vi "FTW-Test-Actor-Stress.vi"() -> (0 "Test Result":errorcluster)   [LabVIEW 2015]
uses:
  src/time/FTW-Time-RelativeTimer.vi
  src/error/FTW-ERR-PrependExplanation.vi
  src/error/FTW-ERR-Ignore.vi
  src/error/FTW-ERR-ThrowError.vi
  src/reflection/FTW-Reflection-Type.vi
  src/error/FTW-ERR-StatusException.vi
  src/error/FTW-ERR-CallChain.vi
  src/string/FTW-STR-ReplaceWhitespace.vi
  src/reflection/FTW-Reflection-Array.vi
  src/error/FTW-ERR-Clear.vi
  src/regex/FTW-Regex-ReplaceAll.vi
  src/json/FTW-JSON-Construct-FromBuffer.vi
  src/json/FTW-JSON-Object-GetElement-String.vi
  src/socket/syncserver/FTW-SyncServer-Construct.vi
  src/json/FTW-JSON-Object-SetElement-String.vi
  src/json/FTW-JSON-Object-GetElement-Bool.vi
  src/json/FTW-JSON-Object-GetElement-Integer.vi
  src/json/FTW-JSON-SerializeAndDestroy.vi
  src/actor/support/FTW-Actor-DynamicLaunchOptions.vi
  src/socket/syncserver/FTW-SyncServer-Await.vi
  src/actor/request/FTW-Request-InterpretResponse.vi
  lib/FTW-KernelFilepath.vi
  src/json/core/FTW-JSON-Core-EncodingFlags.vi
  codegen/xnode/json/fetch/FTW-JSON-Core-GetFlattenedValue.vi
  src/socket/connector/FTW-Connector-Construct.vi
  src/socket/syncserver/FTW-SyncServer-Reply.vi
  src/socket/syncserver/FTW-SyncServer-Destroy.vi
  codegen/xnode/FTW-Dataflow-Synchronizer.xnode
  codegen/xnode/FTW-Actor-Spawn.xnode
  src/core/type/FTW-Type-Actor-Connector.ctl
  codegen/xnode/FTW-JSON-Fetch.xnode
panel:
  out "Actor Lifetimes":dbl[][](graph)
  out "Timeline":cluster{dbl[], i32[]}[](graph)
  in  "Test to Perform":T1(radio)=enum."true 10x10"
  out "Message Times":dbl[][](graph)
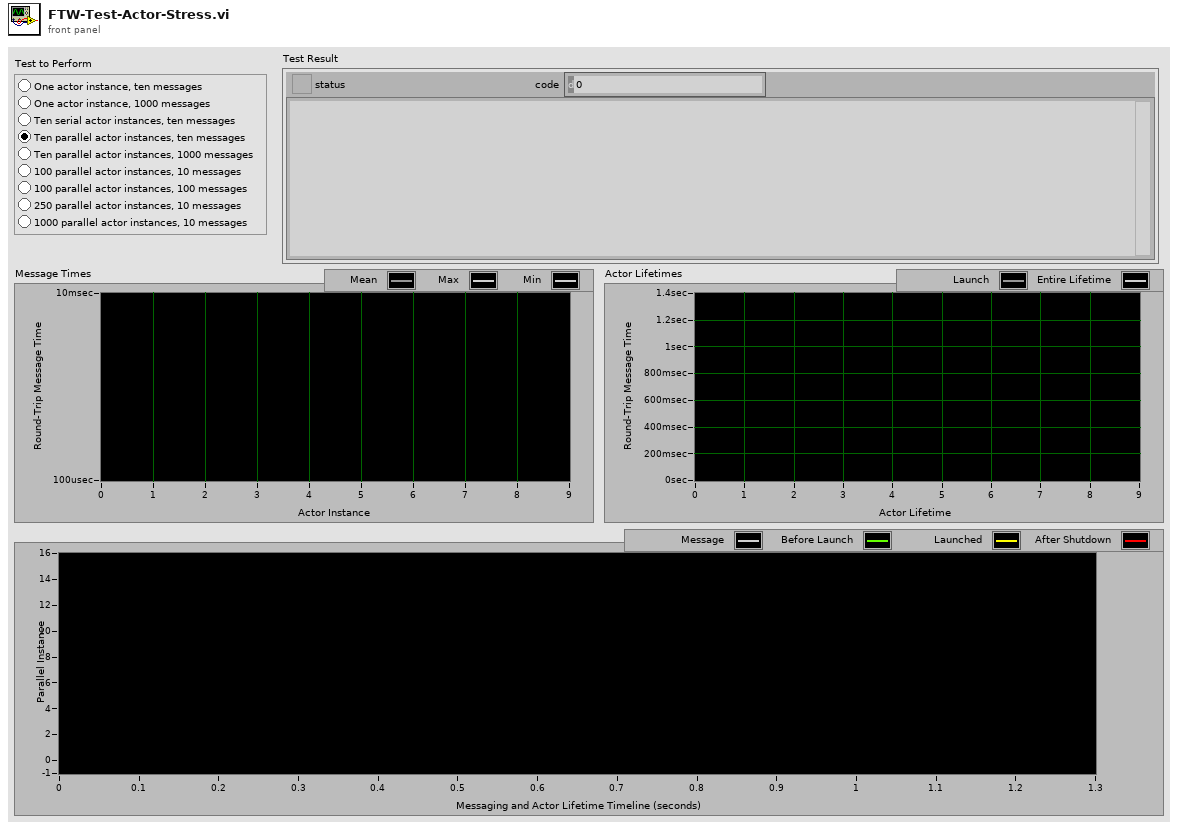
[diagram p1: front panel]
types:
  T1 = enum32{"false 1x10", "false 1x1000", "false 10x10", "true 10x10", "true 10x1000", "true 100x10", "true 100x100", "true 250x10", "true 1000x10"}
  T2 = cluster{"FTW-PrimaryInboxAddress":string, "FTW-InstanceCloneName":string}
  T3 = typedef "FTW-Type-Actor-Connector.ctl" = refnum<data-value>
  T4 = cluster{i32, "High-Resolution Timer":dbl, "Instance Inbox Address":string, "Instance VI Clone Name":string, "High-Resolution Timer":dbl, dbl[], dbl[], "High-Resolution Timer":dbl, "error out out":errorcluster}
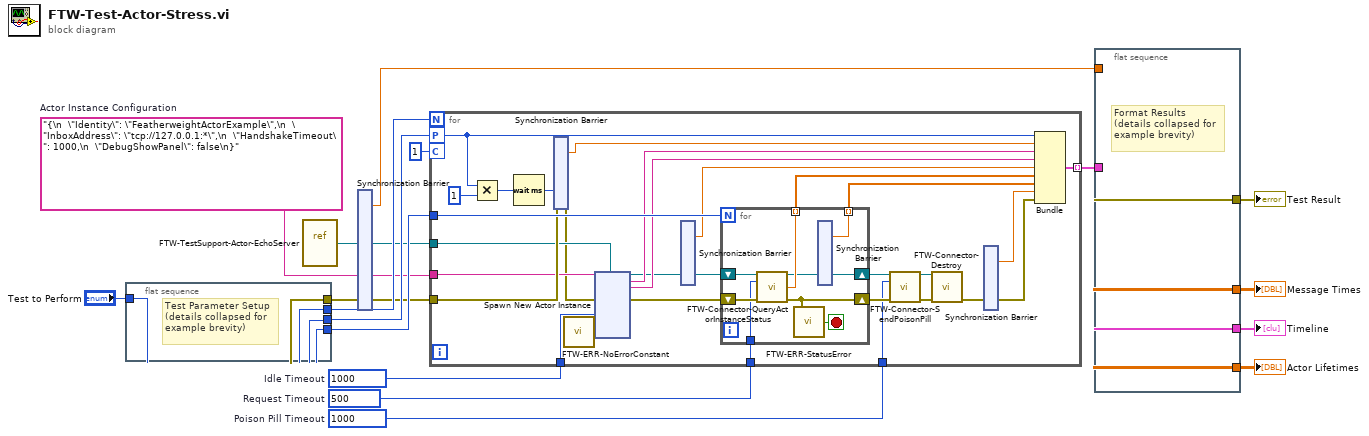
[diagram p0: block diagram]
diagram:
  w1 = 1000  # Poison Pill Timeout
  w2 = 500  # Request Timeout
  w3 = 1000  # Idle Timeout
  w5 = "{\n  \"Identity\": \"FeatherweightActorExample\",\n  \"InboxAddress\": \"tcp://127.0.0.1:*\",\n  \"HandshakeTimeout\": 1000,\n  \"DebugShowPanel\": false\n}"  # Actor Instance Configuration
  n1 = flat-sequence {
    tunnel: "Test to Perform" -> [w21]
    tunnel: [w26] -> w19
    tunnel: [w25] -> w18
    tunnel: [w23] -> w16
    tunnel: [w22] -> w15
    frame #0 {
      w28 = FALSE  # Parallelize?
      # "Test Parameter Setup\n(details collapsed for\nexample brevity)"
      n2 = Format Into String(w21) -> (resulting string=w30:string, error out=w29:errorcluster)  [unwired: 3 in]
      n3 = Scan From String(format string="%s %dx%d", input string=w30, error in=w29, default 1=w28, default 2=0, default 3=0) -> (error out=w22:errorcluster, output 1=w24:bool, output 2=w23:i32, output 3=w25:i32)  [unwired: 1 in, 2 out]
      n4 = Select(t=w23, s=w24, f=1) -> (s? t:f=w26:i32)
    }
  }
  n5 = vi-ref "FTW-TestSupport-Actor-EchoServer.vi"() -> (w17:refnum<vi>)
  n6 = xnode "Synchronization Barrier"(w17, "Synchronized Signal 5"=w5, "Synchronized Signal 8"=w15) -> ("High-Resolution Timer"=w8:dbl, "out"=w9:refnum<vi>, "Actor Instance Configuration out"=w4:string, "error IO out"=w10:errorcluster)  [unwired: 6 in, 1 out]
  n7 = for {
    N: w16 -> [_]
    tunnel: w4 -> [w46]
    tunnel: w10 -> [w55]
    tunnel: w9 -> [w47]
    tunnel: w18 -> [w59]
    workers-P: w19 -> [w36]
    tunnel: [w52] -> w13 mode=indexing
    chunk-C: 1 -> [_]
    tunnel: w3 -> [w41]
    tunnel: w2 -> [w49]
    tunnel: w1 -> [w48]
    n8 = Multiply(x=w36, y=1) -> (x*y=w34:i32)
    n9 = Wait (ms)(milliseconds to wait=w34) -> (millisecond timer value=w37:u32)
    n10 = xnode "Synchronization Barrier"(w37, "Synchronized Signal 1"=w55) -> ("High-Resolution Timer"=w54:dbl, "error IO out out"=w45:errorcluster)  [unwired: 1 in, 2 out]
    n11 = call "FTW-ERR-NoErrorConstant.vi"() -> ("no error"=w42:errorcluster)
    n12 = xnode "Spawn New Actor Instance"("Actor Instance Configuration"=w46, "Actor Instance Interface"=w47, "error in"=w45, "Idle Timeout"=w41, "ErrorIn"=w42) -> ("FTW Actor Connector"=w38:T3, "Instance Inbox Address"=w39:string, "Instance VI Clone Name"=w44:string, "error out"=w43:errorcluster)  [unwired: 1 in]
    n13 = xnode "Synchronization Barrier"("Synchronized Signal 1"=w38) -> ("High-Resolution Timer"=w53:dbl, "FTW Actor Connector out"=w40:T3)  [unwired: 1 in, 1 out]
    n14 = for {
      N: w59 -> [_]
      tunnel: [w271] -> w62 mode=indexing
      shift-right: [w269] -> w51
      shift-left: w40 -> [w275]
      shift-right: [w268] -> w50
      shift-left: w43 -> [w274]
      tunnel: [w272] -> w63 mode=indexing
      tunnel: w49 -> [w267]
      stop <- w273 stop-if-true
      n15 = call "FTW-Connector-QueryActorInstanceStatus.vi"("FTW Actor Connector"=w275, "Timeout"=w267, "error in"=w274) -> ("FTW Actor Connector out"=w270:T3, "Roundtrip Time"=w272:dbl, "error out"=w268:errorcluster)  [unwired: 9 in, 1 out]
      n16 = call "FTW-ERR-StatusError.vi"("error to check"=w268) -> ("Error?"=w273:bool)
      n17 = xnode "Synchronization Barrier"("Synchronized Signal 1"=w270) -> ("High-Resolution Timer"=w271:dbl, "FTW Actor Connector out out"=w269:T3)  [unwired: 1 in, 1 out]
    }
    n18 = call "FTW-Connector-SendPoisonPill.vi"("FTW Actor Connector"=w51, "Timeout"=w48, "error in"=w50) -> ("FTW Actor Connector out"=w61:T3, "error out"=w60:errorcluster)  [unwired: 9 in, 2 out]
    n19 = call "FTW-Connector-Destroy.vi"("FTW Actor Connector"=w61, "error in"=w60) -> ("error out"=w57:errorcluster)  [unwired: 13 in]
    n20 = xnode "Synchronization Barrier"("Synchronized Signal 1"=w57) -> ("High-Resolution Timer"=w58:dbl, "error out out"=w56:errorcluster)  [unwired: 1 in, 1 out]
    n21 = Bundle(w36, "High-Resolution Timer"=w54, "Instance Inbox Address"=w39, "Instance VI Clone Name"=w44, "High-Resolution Timer"=w53, w63, w62, "High-Resolution Timer"=w58, "error out out"=w56) -> (w52:T4)  [unwired: 1 in]
  }
  n22 = flat-sequence {
    tunnel: [w310] -> w14
    tunnel: w13 -> [w305]
    tunnel: [w302] -> w11
    tunnel: w8 -> [w296]
    tunnel: [w292] -> w7
    tunnel: [w284] -> w6
    frame #0 {
      # "Format Results\n(details collapsed for\nexample brevity)"
      n23 = for {
        tunnel: w305 -> [w328] mode=indexing
        tunnel: [w327] -> w309 mode=indexing
        tunnel: [w325] -> _ mode=indexing
        tunnel: [w324] -> w307 mode=concatenating
        tunnel: [w319] -> w300 mode=concatenating
        tunnel: [w314] -> w283 mode=indexing
        tunnel: [w321] -> w294 mode=indexing
        tunnel: [w320] -> w286 mode=indexing
        tunnel: [w318] -> w288 mode=indexing
        tunnel: [w317] -> w290 mode=indexing
        tunnel: [w316] -> w289 mode=indexing
        tunnel: [w315] -> w291 mode=indexing
        tunnel: [w312] -> w282 mode=indexing
        tunnel: "%5$d messages in [%3$5_3psec, %4$5_3psec, %2$5_3psec] for %1$s" ("format string") -> [w311]
        n24 = Unbundle(w328) -> (w321:i32, "High-Resolution Timer"=w314:dbl, "Instance VI Clone Name"=w313:string, "High-Resolution Timer"=w318:dbl, w322:dbl[], w319:dbl[], "High-Resolution Timer"=w320:dbl, "error out out"=w312:errorcluster)  [unwired: 1 out]
        n25 = Bundle(w322) -> (w325:cluster{dbl[]})  [unwired: 1 in]
        n26 = Add Array Elements(numeric array=w322) -> (sum=w326:dbl)
        n27 = Array Size(array=w322) -> (size(s)=w323:i32)
        n28 = Divide(x=w326, y=w323) -> (x/y=w315:dbl)
        n29 = Array Max & Min(array=w322) -> (max value=w317:dbl, min value=w316:dbl)  [unwired: 2 out]
        n30 = Initialize Array(w321, w323) -> (w324:i32[])
        n31 = Format Into String(format string=w311, w313, w317, w316, w315, w323) -> (resulting string=w327:string)  [unwired: 2 in, 1 out]
      }
      n32 = Merge Errors(w282) -> (w281:errorcluster)
      n33 = Subtract(x=w300, y=w296) -> (x-y=w299:dbl[])
      n34 = Subtract(x=w283, y=w296) -> (x-y=w298:dbl[])
      n35 = Subtract(x=w288, y=w296) -> (x-y=w295:dbl[])
      n36 = Subtract(x=w286, y=w296) -> (x-y=w297:dbl[])
      n37 = Subtract(x=w288, y=w283) -> (x-y=w287:dbl[])
      n38 = Subtract(x=w286, y=w283) -> (x-y=w285:dbl[])
      n39 = call "FTW-STR-Array-Delimit.vi"("Array of Strings"=w309, "Delimiter"="\r\n") -> ("Delimited String"=w306:string)  [unwired: 13 in]
      n40 = Build Array(w291, w290, w289) -> (w292:dbl[][])
      n41 = Build Array(w287, w285) -> (w284:dbl[][])
      n42 = Bundle(w299, w307) -> (w304:cluster{dbl[], i32[]})  [unwired: 1 in]
      n43 = Bundle(w298, w294) -> (w303:cluster{dbl[], i32[]})  [unwired: 1 in]
      n44 = Bundle(w295, w294) -> (w293:cluster{dbl[], i32[]})  [unwired: 1 in]
      n45 = Bundle(w297, w294) -> (w301:cluster{dbl[], i32[]})  [unwired: 1 in]
      n46 = call "FTW-ERR-ThrowInfo.vi"("Informational Message"=w306, "error in"=w281) -> ("error out"=w310:errorcluster)  [unwired: 13 in]
      n47 = Build Array(w304, w303, w293, w301) -> (w302:cluster{dbl[], i32[]}[])
    }
  }
  "Test Result" <- w14
  "Message Times" <- w7
  "Timeline" <- w11
  "Actor Lifetimes" <- w6
